vi "Center speed graph cursor on Y.vi"(8 "error in (no error)":errorcluster) -> (0 "error out":errorcluster)   [LabVIEW 2017]
uses:
  Globals/gl_Time series viewer globals.vi
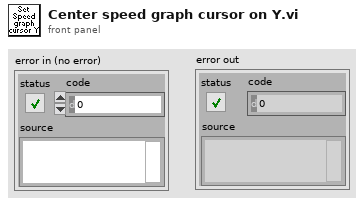
[diagram p1: front panel]
types:
  T1 = typedef "Time series viewer refs.ctl" = cluster{"This VI":refnum<vi>, "Image control":refnum<vi>, "AVI Mode ind":refnum<vi>, "Play":refnum<vi>, "Stop":refnum<vi>, "Back":refnum<vi>, "Scrollbar":refnum<vi>, "Video length info":refnum<vi>, "Expected speed values":refnum<vi>, "Intensity":refnum<vi>, "Path":refnum<vi>, "Selection sliders":refnum<vi>, "Speed Graph ref":refnum<vi>, "Frame rate set (fps)":refnum<vi>, "Channel to load":refnum<vi>, "Number of rows to generate":refnum<vi>, "Colour":refnum<vi>}
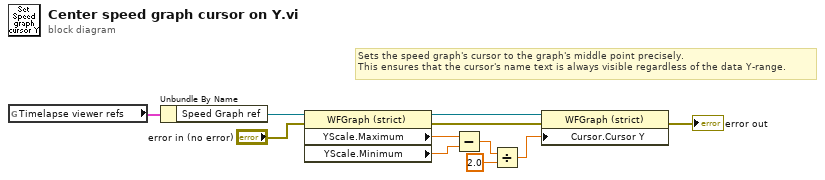
[diagram p0: block diagram]
diagram:
  # "Sets the speed graph's cursor to the graph's middle point precisely.\nThis ensures that the cursor's name text is always visible regardless of the data Y-range."
  n1 = global read "gl_Time series viewer globals.vi" "Timelapse viewer refs"() -> (w9:T1)
  n2 = Unbundle By Name(w9) -> ("Speed Graph ref"=w10:refnum<vi>)
  n3 = property on="Property Node" class="WFGraph (strict)"(reference=w10, error in="error in (no error)") -> (reference out=w8:refnum<vi>, error out=w6:errorcluster, "YScale.Maximum"=w4:dbl, "YScale.Minimum"=w3:dbl)
  n4 = Subtract(x=w4, y=w3) -> (x-y=w2:dbl)
  n5 = Divide(x=w2, y=2.0) -> (x/y=w1:dbl)
  n6 = property on="Property Node" class="WFGraph (strict)"(reference=w8, error in=w6, "Cursor.Cursor Y"=w1) -> (error out=→"error out":errorcluster)  [unwired: 1 out]
